vi "画图片.vi"() -> ()   [LabVIEW 2010]
panel:
  out "图片":picture
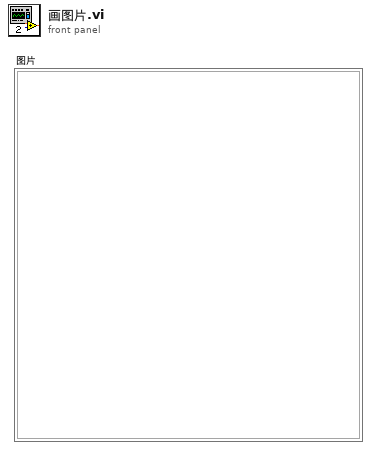
[diagram p1: front panel]
types:
  T1 = cluster{"left":i16, "top":i16, "right":i16, "bottom":i16}
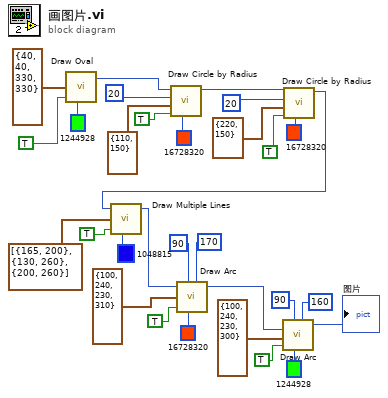
[diagram p0: block diagram]
diagram:
  n1 = call <vilib>:"Draw Oval.vi"("rect"=T1 {"left"=40, "top"=40, "right"=330, "bottom"=330}, "fill?(F)"=TRUE, "color(black)"=u32 1244928) -> ("new picture"=w28:picture)  [unwired: 6 in]
  n2 = call <vilib>:"Draw Circle by Radius.vi"("color(black)"=u32 16728320, "fill?(F)"=TRUE, "pixel center"=cluster{"horizontal":i16, "vertical":i16} {"horizontal"=110, "vertical"=150}, "radius"=i16 20, "picture"=w28) -> ("new picture"=w21:picture)  [unwired: 6 in]
  n3 = call <vilib>:"Draw Circle by Radius.vi"("color(black)"=u32 16728320, "fill?(F)"=TRUE, "pixel center"=cluster{"horizontal":i16, "vertical":i16} {"horizontal"=220, "vertical"=150}, "radius"=i16 20, "picture"=w21) -> ("new picture"=w17:picture)  [unwired: 6 in]
  n4 = call <vilib>:"Draw Multiple Lines.vi"("picture"=w17, "line endpoints"=cluster{"x":i16, "y":i16}[] [{"x"=165, "y"=200}, {"x"=130, "y"=260}, {"x"=200, "y"=260}], "fill?(F)"=TRUE, "color(black)"=u32 1048815) -> ("new picture"=w13:picture)  [unwired: 5 in]
  n5 = call <vilib>:"Draw Arc.vi"("picture"=w13, "start angle[degrees]"=i16 90, "rect"=T1 {"left"=100, "top"=240, "right"=230, "bottom"=310}, "fill?(F)"=TRUE, "color(black)"=u32 16728320, "arc size[degrees]"=i16 170) -> ("new picture"=w10:picture)  [unwired: 3 in]
  n6 = call <vilib>:"Draw Arc.vi"("picture"=w10, "start angle[degrees]"=i16 90, "rect"=T1 {"left"=100, "top"=240, "right"=230, "bottom"=300}, "fill?(F)"=TRUE, "color(black)"=u32 1244928, "arc size[degrees]"=i16 160) -> ("new picture"=→"图片":picture)  [unwired: 3 in]
